vi "Read HostName.vi"(8 "error in (no error)":errorcluster, 11 "CI Project in":refnum<class "CI Project.lvclass">) -> (0 "error out":errorcluster, 2 "HostName":string, 3 "CI Project out":refnum<class "CI Project.lvclass">)   [LabVIEW 2014, in "CI Project.lvclass"]
uses:
  CI Project.lvclass
  CI Project.lvclass/CI Project.ctl
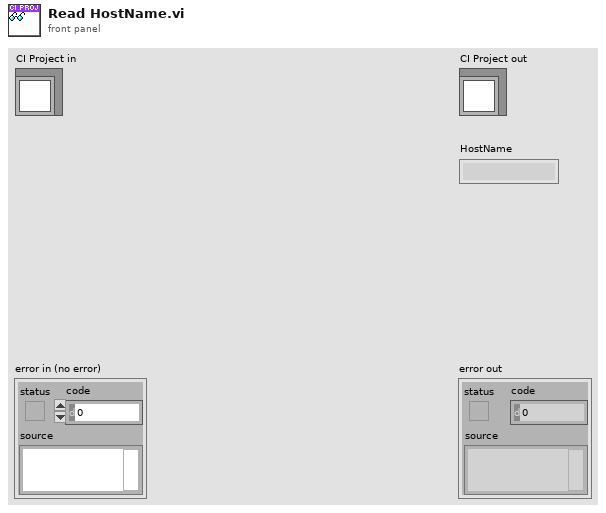
[diagram p1: front panel]
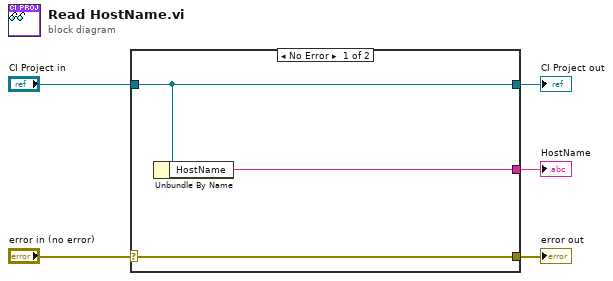
[diagram p0: block diagram]
diagram:
  n1 = case shown="No Error" "error in (no error)" {
    selector: "error in (no error)" -> [w8 w9]
    tunnel: [w8 w9] -> w4
    tunnel: [w7 w10] -> w2
    tunnel: "CI Project in" -> [w7 w10]
    tunnel: [w6 _] -> w1
    frame No Error {
      n2 = Unbundle By Name(w7) -> ("HostName"=w6:string)
    }
    frame Error {
    }
  }
  "error out" <- w4
  "CI Project out" <- w2
  "HostName" <- w1
